vi "InitListener.vi"(8 "error in (no error)":errorcluster, 11 "WebSocket in":refnum<class "WebSocket.lvclass">) -> (0 "error out":errorcluster, 3 "WebSocket out":refnum<class "WebSocket.lvclass">)   [LabVIEW 2019, in "WebSocket.lvlib" / "WebSocket.lvclass"]
uses:
  WebSocket.lvclass
  WebSocket.lvclass/WebSocket.ctl
  <vilib>/MediaMongrels Ltd/WebSockets/Sockets/VISA TCP Listener/VISA TCP Listener.lvclass
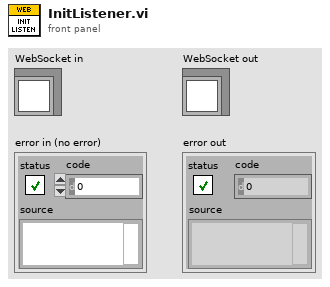
[diagram p1: front panel]
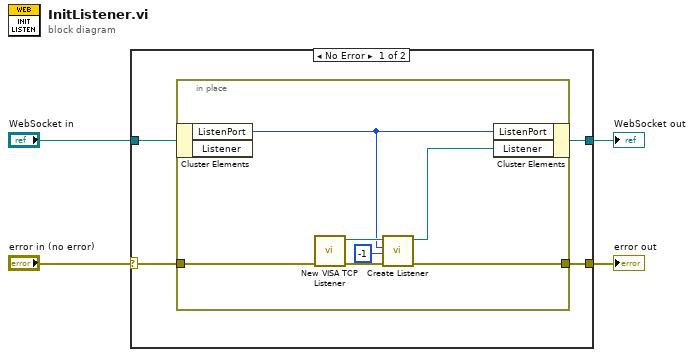
[diagram p0: block diagram]
diagram:
  n1 = case shown="No Error" "error in (no error)" {
    selector: "error in (no error)" -> [w7 w17]
    tunnel: [w6 w17] -> w3
    tunnel: [w5 w16] -> w1
    tunnel: "WebSocket in" -> [w8 w16]
    frame No Error {
      n2 = in-place {
        in-place-border: w7 -> [w11]
        in-place-border: [w10] -> w6
        n3 = in-place-cluster #1(w8) -> ("ListenPort"=w12:u16)  [unwired: 1 out]
        n4 = call <vilib>:"New VISA TCP Listener.vi"("error in (no error)"=w11) -> ("error out"=w14:errorcluster, "VISA TCP Listener out"=w15:refnum<class "VISA TCP Listener.lvclass">)  [unwired: 9 in]
        n5 = call-dynamic "Create Listener.vi"("error in (no error)"=w14, "timeout ms (5000)"=-1, "Port"=w12, "VISA TCP Listener in"=w15) -> ("error out"=w10:errorcluster, "VISA TCP Listener out"=w13:refnum<class "VISA TCP Listener.lvclass">)  [unwired: 6 in]
        n6 = in-place-cluster #1("ListenPort"=w12, "Listener"=w13) -> (w5:refnum<class "WebSocket.lvclass">)
      }
    }
    frame Error {
    }
  }
  "error out" <- w3
  "WebSocket out" <- w1
